vi "Send Calibrations+Settings to Dash.vi"   [LabVIEW 2014]
uses:
  Global Variables/Calibrations.vi
  <vilib>/Rock Robotics/Network Tables/SD Write Numeric Array.vi
  Global Variables/Settings.vi
types:
  T1 = cluster{"proportional gain (Kc)":dbl, "integral time (Ti, min)":dbl, "derivative time (Td, min)":dbl, "Maximum Value":dbl, "Minimum Value":dbl, "epsilon":dbl}
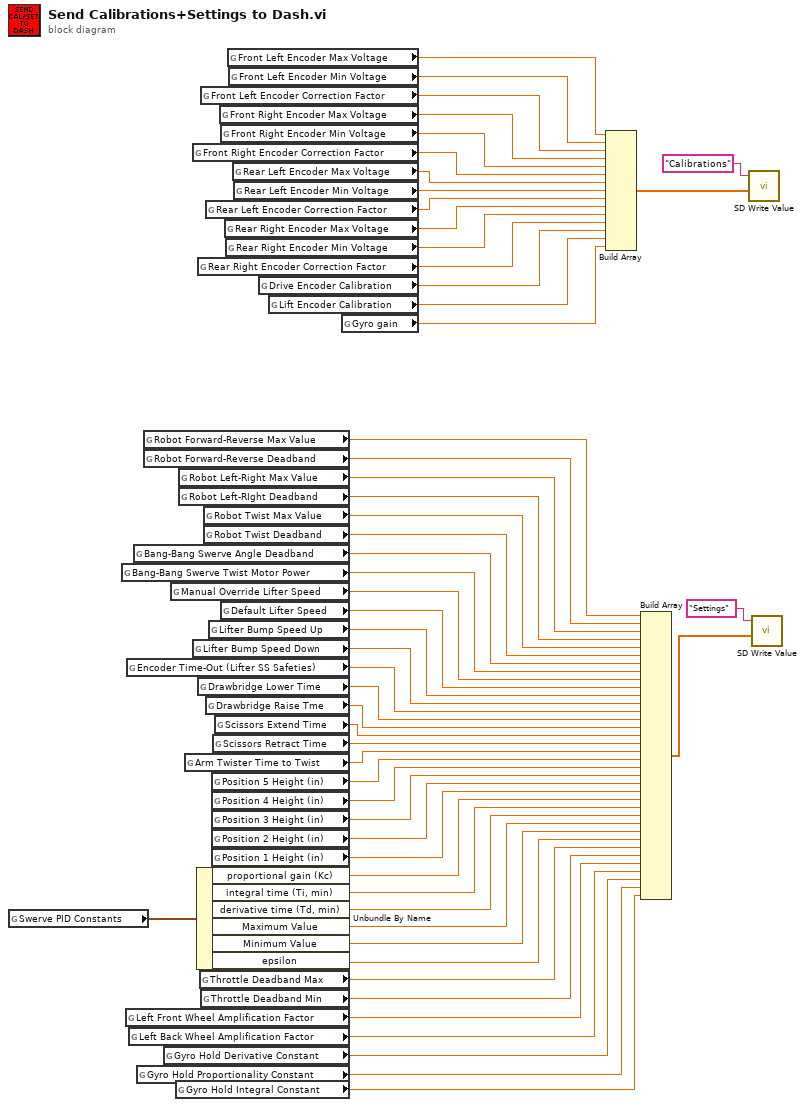
[diagram p0: block diagram]
diagram:
  n1 = global read "Settings.vi" "Swerve PID Constants"() -> (w38:T1)
  n2 = global read "Settings.vi" "Bang-Bang Swerve Twist Motor Power"() -> (w30:dbl)
  n3 = global read "Settings.vi" "Left Front Wheel Amplification Factor"() -> (w6:dbl)
  n4 = global read "Settings.vi" "Encoder Time-Out (Lifter SS Safeties)"() -> (w25:dbl)
  n5 = global read "Settings.vi" "Left Back Wheel Amplification Factor"() -> (w5:dbl)
  n6 = global read "Settings.vi" "Bang-Bang Swerve Angle Deadband"() -> (w31:dbl)
  n7 = global read "Settings.vi" "Gyro Hold Proportionality Constant"() -> (w3:dbl)
  n8 = global read "Settings.vi" "Robot Forward-Reverse Max Value"() -> (w37:dbl)
  n9 = global read "Settings.vi" "Robot Forward-Reverse Deadband"() -> (w36:dbl)
  n10 = global read "Settings.vi" "Gyro Hold Derivative Constant"() -> (w4:dbl)
  n11 = global read "Settings.vi" "Manual Override Lifter Speed"() -> (w29:dbl)
  n12 = global read "Settings.vi" "Gyro Hold Integral Constant"() -> (w2:dbl)
  n13 = global read "Settings.vi" "Robot Left-Right Max Value"() -> (w35:dbl)
  n14 = global read "Settings.vi" "Robot Left-RIght Deadband"() -> (w34:dbl)
  n15 = global read "Settings.vi" "Arm Twister Time to Twist"() -> (w22:dbl)
  n16 = global read "Calibrations.vi" "Front Right Encoder Correction Factor"() -> (w51:dbl)
  n17 = global read "Settings.vi" "Lifter Bump Speed Down"() -> (w26:dbl)
  n18 = Unbundle By Name(w38) -> ("proportional gain (Kc)"=w15:dbl, "integral time (Ti, min)"=w14:dbl, "derivative time (Td, min)"=w13:dbl, "Maximum Value"=w12:dbl, "Minimum Value"=w11:dbl, "epsilon"=w9:dbl)
  n19 = global read "Calibrations.vi" "Rear Right Encoder Correction Factor"() -> (w45:dbl)
  n20 = global read "Settings.vi" "Drawbridge Lower Time"() -> (w24:dbl)
  n21 = global read "Settings.vi" "Throttle Deadband Max"() -> (w8:dbl)
  n22 = global read "Calibrations.vi" "Front Left Encoder Correction Factor"() -> (w54:dbl)
  n23 = global read "Settings.vi" "Throttle Deadband Min"() -> (w7:dbl)
  n24 = global read "Settings.vi" "Robot Twist Max Value"() -> (w33:dbl)
  n25 = global read "Settings.vi" "Robot Twist Deadband"() -> (w32:dbl)
  n26 = global read "Calibrations.vi" "Rear Left Encoder Correction Factor"() -> (w48:dbl)
  n27 = global read "Settings.vi" "Drawbridge Raise Tme"() -> (w23:dbl)
  n28 = global read "Settings.vi" "Lifter Bump Speed Up"() -> (w27:dbl)
  n29 = global read "Settings.vi" "Position 5 Height (in)"() -> (w20:dbl)
  n30 = global read "Settings.vi" "Position 4 Height (in)"() -> (w19:dbl)
  n31 = global read "Settings.vi" "Position 3 Height (in)"() -> (w18:dbl)
  n32 = global read "Settings.vi" "Position 2 Height (in)"() -> (w17:dbl)
  n33 = global read "Settings.vi" "Position 1 Height (in)"() -> (w16:dbl)
  n34 = global read "Settings.vi" "Scissors Retract Time"() -> (w21:dbl)
  n35 = global read "Settings.vi" "Scissors Extend Time"() -> (w10:dbl)
  n36 = global read "Calibrations.vi" "Front Right Encoder Max Voltage"() -> (w53:dbl)
  n37 = global read "Calibrations.vi" "Front Right Encoder Min Voltage"() -> (w52:dbl)
  n38 = global read "Settings.vi" "Default Lifter Speed"() -> (w28:dbl)
  n39 = global read "Calibrations.vi" "Rear Right Encoder Max Voltage"() -> (w47:dbl)
  n40 = global read "Calibrations.vi" "Rear Right Encoder Min Voltage"() -> (w46:dbl)
  n41 = global read "Calibrations.vi" "Front Left Encoder Max Voltage"() -> (w56:dbl)
  n42 = global read "Calibrations.vi" "Front Left Encoder Min Voltage"() -> (w55:dbl)
  n43 = global read "Calibrations.vi" "Rear Left Encoder Max Voltage"() -> (w49:dbl)
  n44 = global read "Calibrations.vi" "Rear Left Encoder Min Voltage"() -> (w50:dbl)
  n45 = global read "Calibrations.vi" "Drive Encoder Calibration"() -> (w44:dbl)
  n46 = global read "Calibrations.vi" "Lift Encoder Calibration"() -> (w43:dbl)
  n47 = global read "Calibrations.vi" "Gyro gain"() -> (w42:dbl)
  n48 = Build Array(w56, w55, w54, w53, w52, w51, w49, w50, w48, w47, w46, w45, w44, w43, w42) -> (w41:dbl[])
  n49 = Build Array(w37, w36, w35, w34, w33, w32, w31, w30, w29, w28, w27, w26, w25, w24, w23, w10, w21, w22, w20, w19, w18, w17, w16, w15, w14, w13, w12, w11, w9, w8, w7, w6, w5, w4, w3, w2) -> (w1:dbl[])
  n50 = call-poly <vilib>:"SD Write Value.vi"("Numeric Array"=w41, "Name"="Calibrations") -> ()  [unwired: 8 in, 2 out]
  n51 = call-poly <vilib>:"SD Write Value.vi"("Numeric Array"=w1, "Name"="Settings") -> ()  [unwired: 8 in, 2 out]
